vi "Rising Edge.vi"(7 "Rise/Fall? (Rise = true)":bool=TRUE, 11 "signal":bool) -> (3 "edge?":bool)   [LabVIEW 2025]
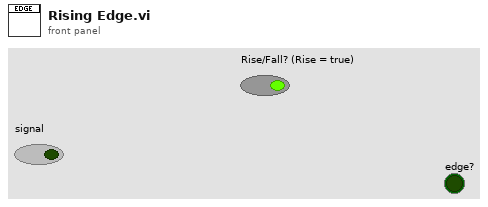
[diagram p1: front panel]
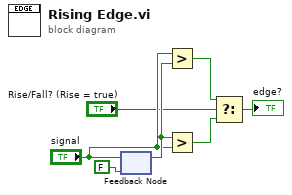
[diagram p0: block diagram]
diagram:
  n1 = feedback-in #1("signal") -> ()
  n2 = feedback #1(FALSE ("signal")) -> (w5:bool)
  n3 = Greater?(x="signal", y=w5) -> (0:w1:bool)
  n4 = Greater?(x=w5, y="signal") -> (0:w7:bool)
  n5 = Select(t=w1, s="Rise/Fall? (Rise = true)", f=w7) -> (s? t:f=→"edge?":bool)
